vi "Measurement UI.vi"() -> ()   [LabVIEW 2024, in "PMIC_Efficiency_DMM.lvlib"]
uses:
  PMIC_Efficiency_DMM.lvlib
  measurementlink-labview-examples-2.0.0.1/NI-DMM Measurement/NIDmmMeasurement/ResolutionInDigits.ctl
  measurementlink-labview-examples-2.0.0.1/NI-DMM Measurement/NIDmmMeasurement/NIDmmMeasurement.lvlib
panel:
  out "Iin":dbl[](graph)
  out "Iout":dbl[](graph)
  out "Vin":dbl[](graph)
  out "Efficiency":cluster{dbl[], dbl[]}(graph) caption="DUT Efficiency (%) vs. Load Current (A)"
  in  "Configurations":enum32{"Settings"}(tab)
  in  "Vin Pin Name":string(combo)
  in  "Source Voltage Level (V)":dbl=3.0 format="%#_6p"
  in  "Source Current Limit (A)":dbl=1.0 format="%#_6p"
  in  "Eload Pin Name":string(combo)
  in  "Load Voltage Limit (V)":dbl=5.0
  in  "Points":i32=10 min=1
  in  "Current Load Level Start":dbl=0.1 min=0.0 step=0.1
  in  "Current Load Level Stop":dbl=1.0 caption="Current load level stop" min=0.0 step=0.1
  in  "Vout Pin Name":string(combo)
  in  "Range":dbl=10.0 format="%.2f"
  in  "Resolution in Digits":T1=enum."5 1/2"
  out "Vout":dbl[](graph)
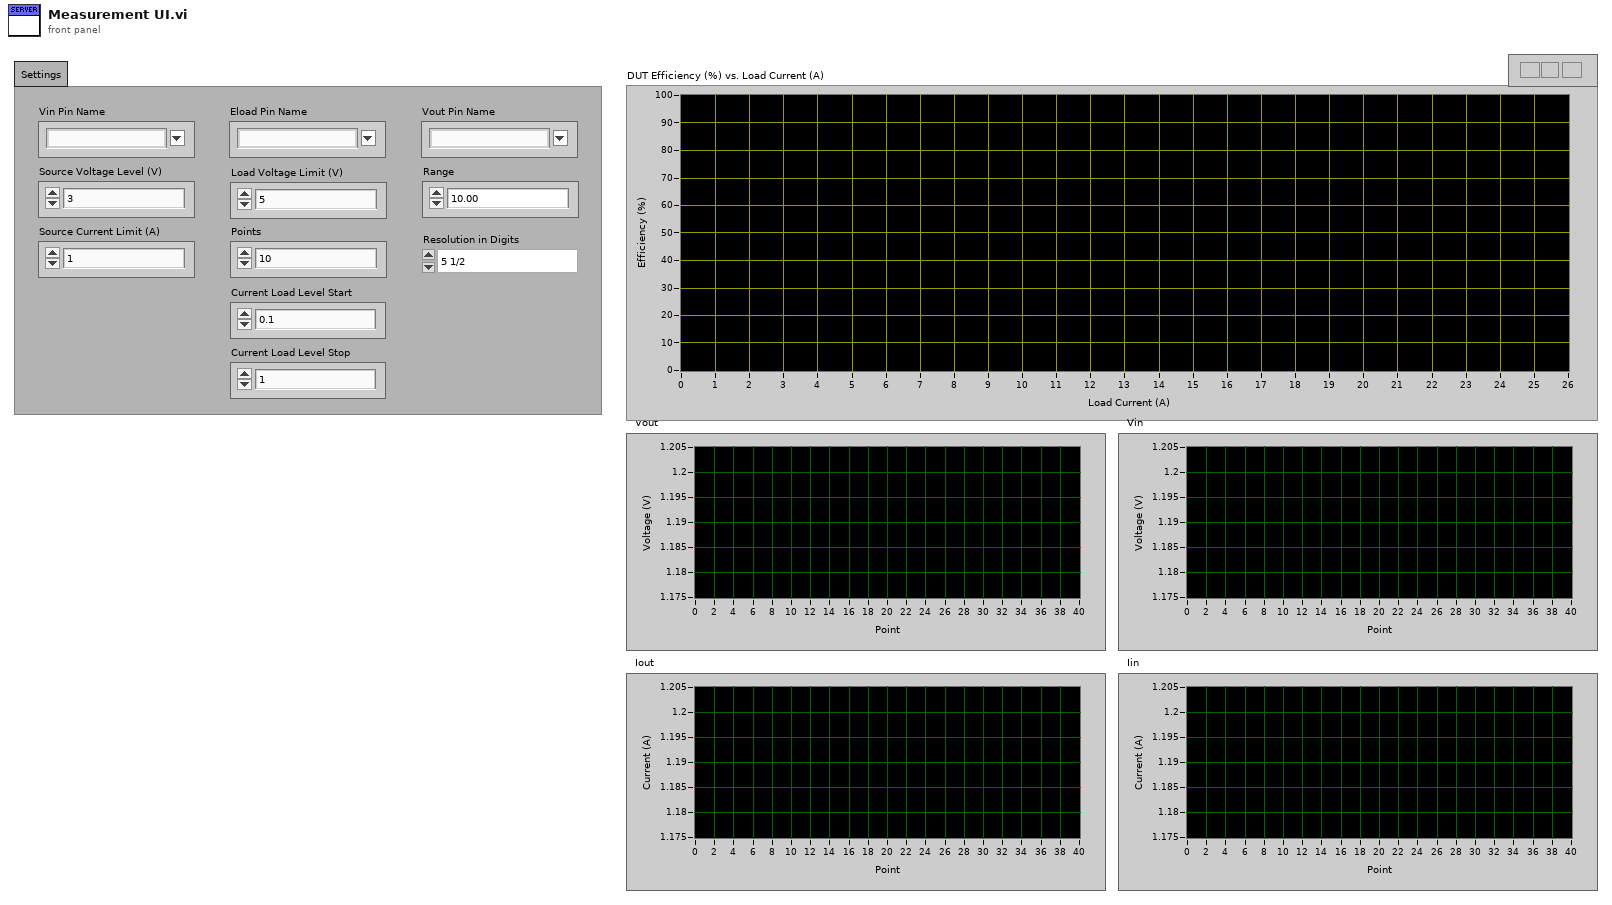
[diagram p1: front panel]
types:
  T1 = typedef "NIDmmMeasurement.lvlib/ResolutionInDigits.ctl" = enum32{"3 1/2", "4 1/2", "5 1/2", "6 1/2", "7 1/2"}
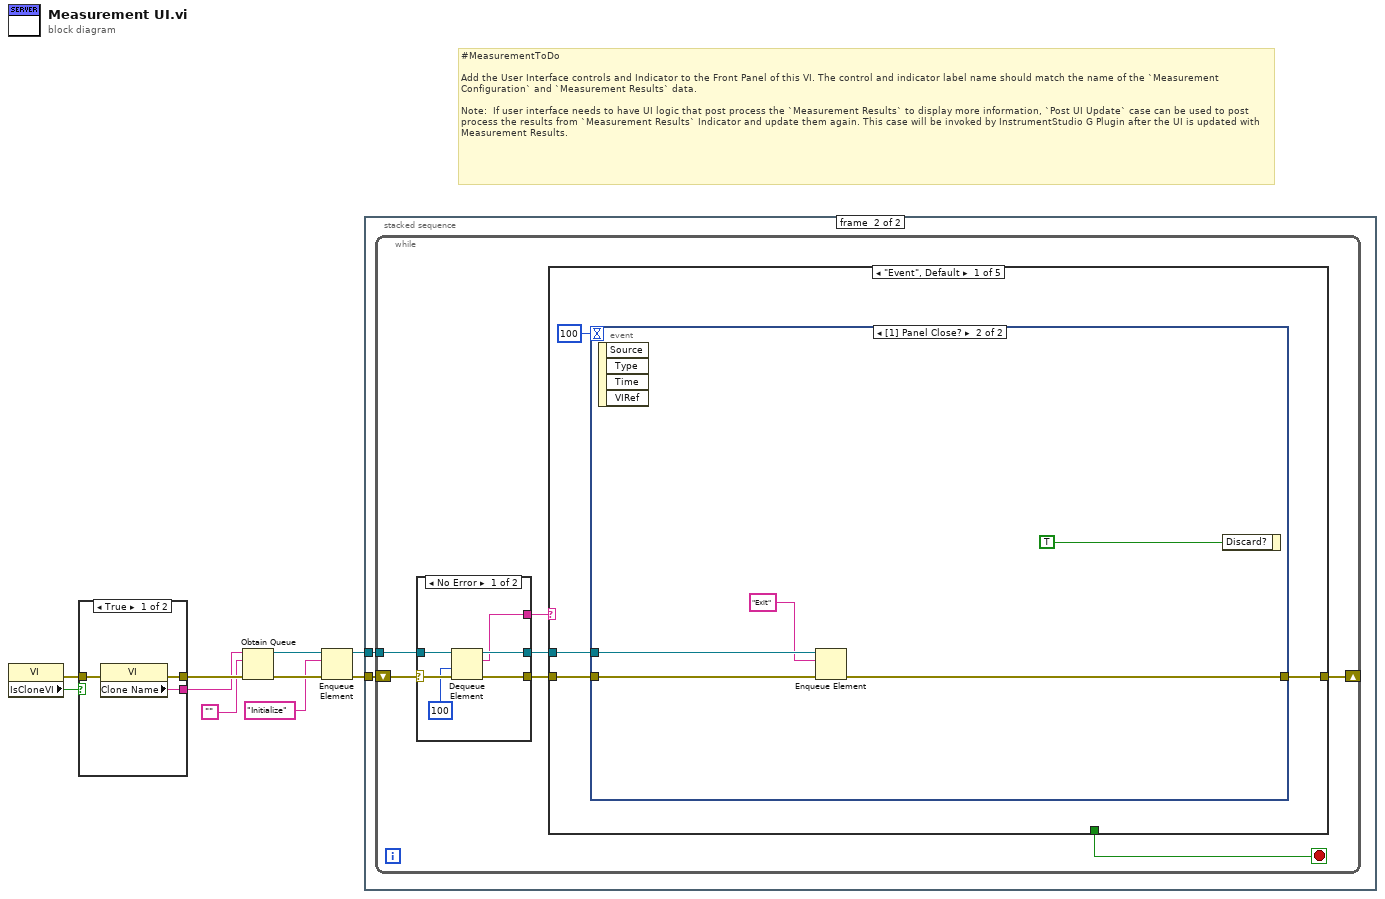
[diagram p0: block diagram]
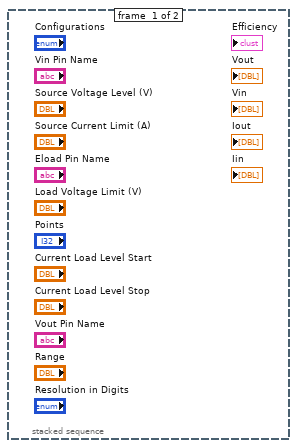
[diagram p2: hidden frame]
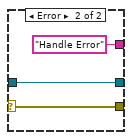
[diagram p3: hidden frame]
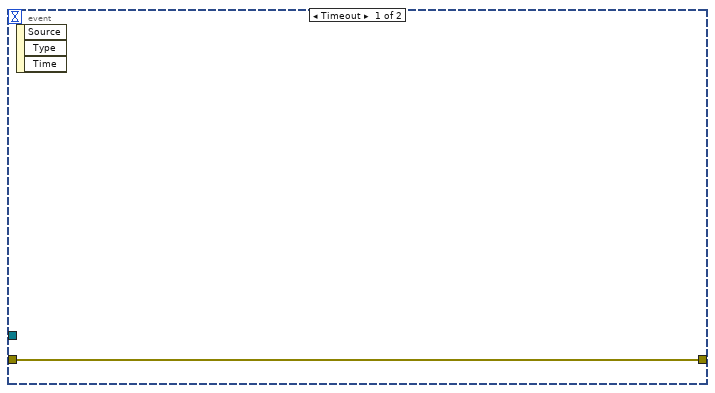
[diagram p4: hidden frame]
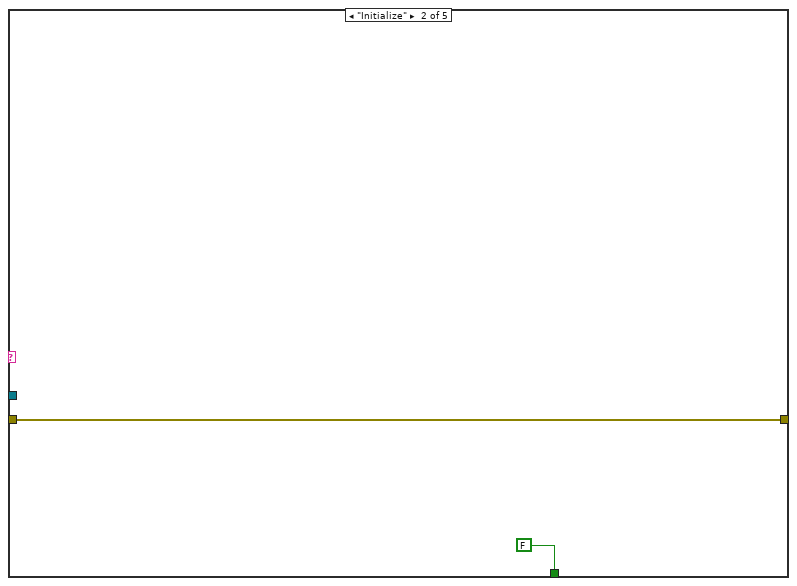
[diagram p5: hidden frame]
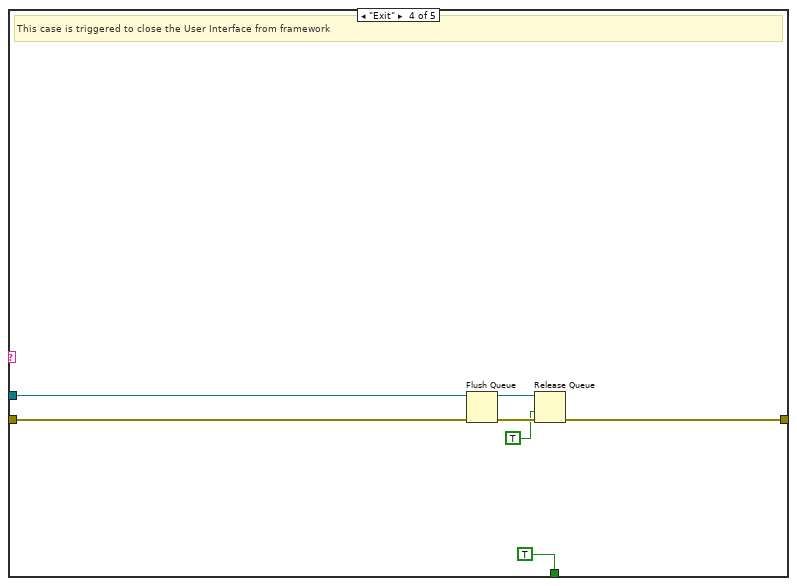
[diagram p7: hidden frame]
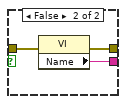
[diagram p9: hidden frame]
diagram:
  # "#MeasurementToDo  \n\nAdd the User Interface controls and Indicator to the Front Panel of this VI. The control and indicator label name should match the name of the `Measurement Configuration` and `Measurement Results` data.\n\nNote:  If user interface needs to have UI logic that post process the `Measurement Results` to display more information, `Post UI Update` case can be used to post process the results from `Measurement Results` Indicator and update them again. This case will be invoked by InstrumentStudio G Plugin after the UI is updated with Measurement Results."
  n1 = property class="VI"() -> (error out=w1:errorcluster, "IsCloneVI"=w2:bool)  [unwired: 2 in, 1 out]
  n2 = case shown="True" w2 {
    tunnel: [w13 w16] -> w10
    tunnel: [w12 w15] -> w9
    tunnel: w1 -> [w11 w14]
    frame True {
      n3 = property class="VI"(error in=w11) -> (error out=w13:errorcluster, "Clone Name"=w12:string)  [unwired: 1 in, 1 out]
    }
    frame False {
      n4 = property class="VI"(error in=w14) -> (error out=w16:errorcluster, "Name"=w15:string)  [unwired: 1 in, 1 out]
    }
  }
  n5 = Obtain Queue(name (unnamed)=w9, element data type="", error in (no error)=w10) -> (queue out=w6:refnum<queue>, error out=w8:errorcluster)  [unwired: 2 in, 1 out]
  n6 = Enqueue Element(queue=w6, element="Initialize", error in (no error)=w8) -> (queue out=w5:refnum<queue>, error out=w7:errorcluster)  [unwired: 1 in, 1 out]
  n7 = stacked-sequence {
    tunnel: w7 -> [_ w18]
    tunnel: w5 -> [_ w17]
    frame #0 {
    }
    frame #1 {
      n8 = while {
        shift-right: [w20] -> _
        shift-left: w18 -> [w25]
        tunnel: w17 -> [w23]
        stop <- w19 stop-if-true
        n9 = case shown="No Error" w25 {
          selector: w25 -> [w31 w34]
          tunnel: [w30 w34] -> w24
          tunnel: w23 -> [w29 w33]
          tunnel: [w28 w33] -> w22
          tunnel: [w27 "Handle Error"] -> w21
          frame No Error {
            n10 = Dequeue Element(queue=w29, timeout in ms (-1)=100, error in (no error)=w31) -> (queue out=w28:refnum<queue>, element=w27:string, error out=w30:errorcluster)  [unwired: 1 out]
          }
          frame Error {
          }
        }
        n11 = case shown="\"Event\", Default" w21 {
          tunnel: w24 -> [w37 w46 w47 w54 w55]
          tunnel: w22 -> [w35 _ _ w52 _]
          tunnel: [w38 w46 w47 w49 w55] -> w20
          tunnel: [_ FALSE _ TRUE _] -> w19
          frame "Event", Default {
            n12 = event shown="[1] Panel Close?" {
              selector: _ -> [_ _]
              dyn-events: _ -> [_ _]
              timeout: 100 -> [_ _]
              tunnel: [w39 w42] -> w38
              tunnel: w37 -> [w39 w43]
              tunnel: w35 -> [_ w41]
              event Timeout {
                n13 = event-data() -> ()  [unwired: 1 in, 3 out]
              }
              event Panel Close? {
                n14 = event-data() -> ()  [unwired: 1 in, 4 out]
                n15 = Enqueue Element(queue=w41, element="Exit", error in (no error)=w43) -> (error out=w42:errorcluster)  [unwired: 1 in, 2 out]
                n16 = event-data("Discard?"=TRUE) -> ()  [unwired: 1 in, 1 out]
              }
            }
          }
          frame "Initialize" {
          }
          frame "Post UI Update" {
            # "This case will be triggered, after framework updates the User interface with result values."
          }
          frame "Exit" {
            # "This case is triggered to close the User Interface from framework"
            n17 = Flush Queue(queue=w52, error in (no error)=w54) -> (queue out=w51:refnum<queue>, error out=w50:errorcluster)  [unwired: 1 out]
            n18 = Release Queue(queue=w51, force destroy? (F)=TRUE, error in (no error)=w50) -> (error out=w49:errorcluster)  [unwired: 2 out]
          }
          frame "Handle Error" {
          }
        }
      }
    }
  }
